vi "TopBar.vi"() -> ()   [LabVIEW 2010]
uses:
  <vilib>/Utility/miscctls.llb/LVPointTypeDef.ctl
panel:
  in  "stop":bool
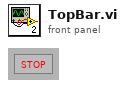
[diagram p1: front panel]
types:
  T1 = typedef "LVPointTypeDef.ctl" = cluster{"Horizontal":i16, "Vertical":i16}
  T2 = typedef "LVRectTypeDef.ctl" = cluster{"left":i16, "top":i16, "right":i16, "bottom":i16}
  T3 = typedef "LVAllMonitorsDisplayTypeDef.ctl" = cluster{"Bounds":cluster{"Left":i16, "Top":i16, "Right":i16, "Bottom":i16}, "Depth":i16}[]
  T4 = cluster{"Bounds":cluster{"Left":i16, "Top":i16, "Right":i16, "Bottom":i16}, "Depth":i16}
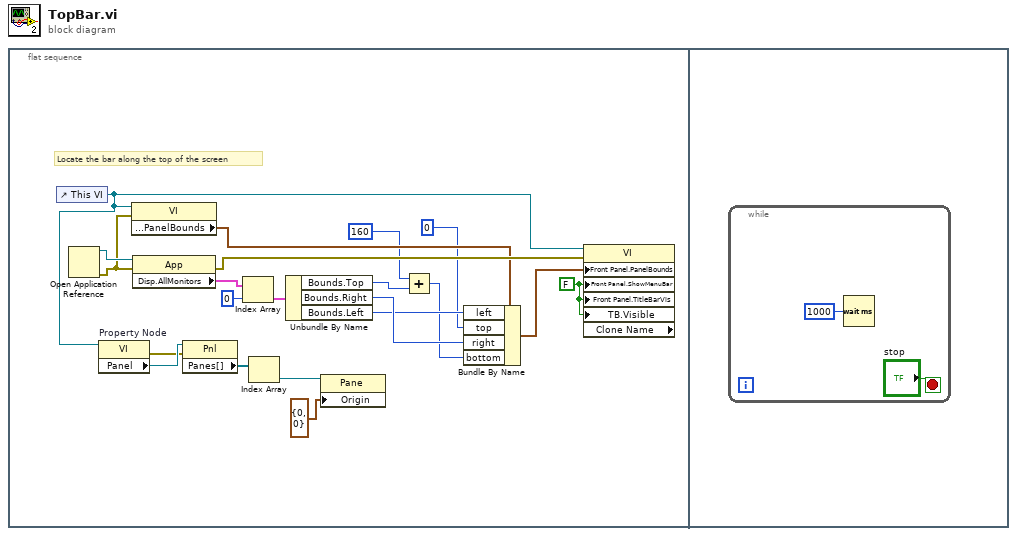
[diagram p0: block diagram]
diagram:
  n1 = flat-sequence {
    frame #0 {
      w2 = FALSE ("Front Panel Window:Show Menu Bar")
      # "Locate the bar along the top of the screen"
      n2 = control-ref of="This VI"() -> (w4:refnum<vi>)
      n3 = Open Application Reference() -> (0:w13:errorcluster, 3:w14:refnum<vi>)  [unwired: 4 in]
      n4 = property on="Property Node" class="VI"(reference=w4) -> (error out=w8:errorcluster, "Panel"=w9:refnum<vi>)  [unwired: 1 in, 1 out]
      n5 = property class="VI"(reference=w4, error in=w13) -> ("Front Panel.PanelBounds"=w10:T2)  [unwired: 2 out]
      n6 = property class="App"(reference=w14, error in=w13) -> (error out=w18:errorcluster, "Disp.AllMonitors"=w20:T3)  [unwired: 1 out]
      n7 = property class="Pnl"(reference=w9, error in=w8) -> ("Panes[]"=w7:refnum<vi>[])  [unwired: 2 out]
      n8 = Index Array(array=w20, index=0) -> (element=w21:T4)
      n9 = Index Array "Index Array"(array=w7) -> (element=w6:refnum<vi>)  [unwired: 1 in]
      n10 = Unbundle By Name(w21) -> ("Bounds.Top"=w12:i16, "Bounds.Right"=w16:i16, "Bounds.Left"=w15:i16)
      n11 = property class="Pane"(reference=w6, "Origin"=T1 {"Horizontal"=0, "Vertical"=0}) -> ()  [unwired: 1 in, 2 out]
      n12 = Add(x=i16 160, y=w12) -> (x+y=w11:i16)
      n13 = Bundle By Name(cluster=w10, "left"=w15, "top"=i16 0, "right"=w16, "bottom"=w11) -> (w17:T2)
      n14 = property on="Property Node" class="VI" props=["Front Panel.PanelBounds", "Front Panel.ShowMenuBar", "Front Panel.TitleBarVis", "TB.Visible", "Clone Name"](reference=w4, error in=w18, "Front Panel.PanelBounds"=w17, "Front Panel.ShowMenuBar"=w2, "Front Panel.TitleBarVis"=w2, "TB.Visible"=w2) -> ()  [unwired: 3 out]
    }
    frame #1 {
      n15 = while {
        stop <- "stop" stop-if-true
        n16 = Wait (ms)(milliseconds to wait=u32 1000) -> ()  [unwired: 1 out]
      }
    }
  }
